vi "SubVI_ControlIntakeLift_Teleop.vi"(11 "Open/close Intake":bool) -> ()   [LabVIEW 2017]
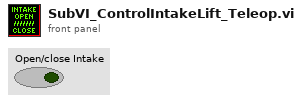
[diagram p1: front panel]
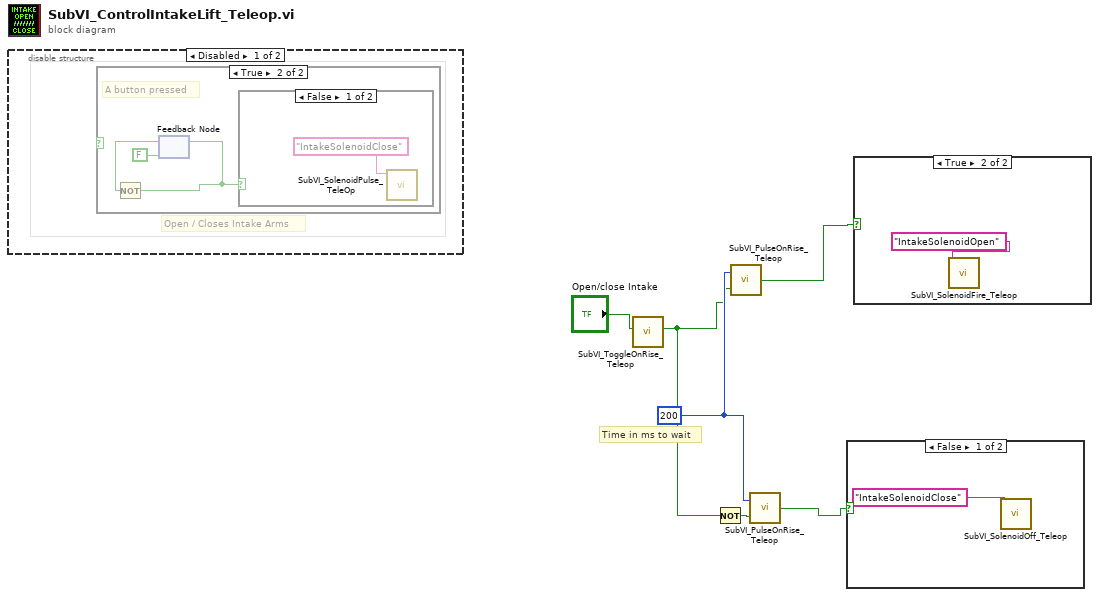
[diagram p0: block diagram]
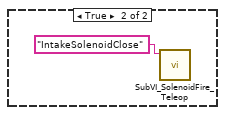
[diagram p2: hidden frame]
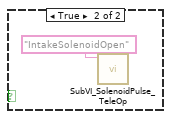
[diagram p4: hidden frame]
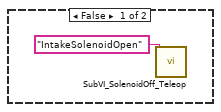
[diagram p6: hidden frame]
diagram:
  w3 = 200 ("Number of milliseconds to wait.\n~20ms precision.")
  # "Time in ms to wait"
  n1 = disable-structure shown="Disabled" {
    frame Disabled {
      # "Open / Closes Intake Arms"
      n2 = case shown="True" {
        selector: _ -> [_ _]
        frame False {
        }
        frame True {
          # "A button pressed"
          n3 = feedback #1(FALSE) -> (w8:bool)
          n4 = Not(x=w8) -> (.not. x?=w7:bool)
          n5 = feedback-in #1(w7) -> ()
          n6 = case shown="False" w7 {
            frame False {
              n7 = call "SubVI_SolenoidPulse_TeleOp.vi"("Solenoid"="IntakeSolenoidClose") -> ()  [unwired: 10 in, 1 out]
            }
            frame True {
              n8 = call "SubVI_SolenoidPulse_TeleOp.vi"("Solenoid"="IntakeSolenoidOpen") -> ()  [unwired: 10 in, 1 out]
            }
          }
        }
      }
    }
    frame Enabled {
    }
  }
  n9 = call "SubVI_ToggleOnRise_Teleop.vi"("Input"="Open/close Intake") -> ("toggled"=w1:bool)  [unwired: 10 in]
  n10 = Not(x=w1) -> (.not. x?=w5:bool)
  n11 = call "SubVI_PulseOnRise_Teleop.vi"("Input"=w1, "Number of milliseconds to wait.\n~20ms precision."=w3) -> ("RisingPulse"=w6:bool)
  n12 = call "SubVI_PulseOnRise_Teleop.vi"("Input"=w5, "Number of milliseconds to wait.\n~20ms precision."=w3) -> ("RisingPulse"=w4:bool)
  n13 = case shown="False" w4 {
    frame False {
      n14 = call "SubVI_SolenoidOff_Teleop.vi"("Solenoid"="IntakeSolenoidClose") -> ()  [unwired: 11 in]
    }
    frame True {
      n15 = call "SubVI_SolenoidFire_Teleop.vi"("Solenoid"="IntakeSolenoidClose") -> ()  [unwired: 11 in]
    }
  }
  n16 = case shown="True" w6 {
    frame False {
      n17 = call "SubVI_SolenoidOff_Teleop.vi"("Solenoid"="IntakeSolenoidOpen") -> ()  [unwired: 11 in]
    }
    frame True {
      n18 = call "SubVI_SolenoidFire_Teleop.vi"("Solenoid"="IntakeSolenoidOpen") -> ()  [unwired: 11 in]
    }
  }
